vi "EulerIntegrator.vi"(1 "xDot":dbl, 5 "dt":dbl, 13 "xInitial":dbl) -> (21 "x":dbl)   [LabVIEW 2012]
panel:
  # "Euler Integrator:  x(k+1) = x(k) + xDot(k) * dt"
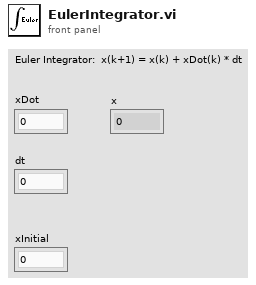
[diagram p1: front panel]
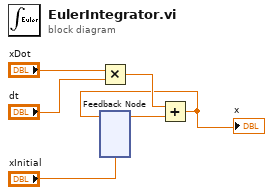
[diagram p0: block diagram]
diagram:
  n1 = Multiply(x="xDot", y="dt") -> (x*y=w4:dbl)
  n2 = feedback #1("xInitial") -> (w2:dbl)
  n3 = Add(x=w4, y=w2) -> (x+y=w1:dbl)
  "x" <- w1
  n4 = feedback-in #1(w1) -> ()
